vi "TimingTest.vi"() -> ()   [LabVIEW 2017]
uses:
  9d5949f9-07ca-45c6-940a-2e3a62ca42df.vi
  <vilib>/express/express analysis/Spectral/Block/exnSpectralBlock spectral measurements RMS poly.vi
  <vilib>/express/express analysis/Spectral/Block/exnSpectralBlock spectral measurements RMS DDT.vi
  <vilib>/express/express analysis/Spectral/XNode/ExpressSpectralMeasurementsBlockNode.xnode
panel:
  in  "100 Hz high-pass":bool
  out "Waveform Graph 2":dynamicdata(graph)
  out "Waveform Graph":dynamicdata(graph)
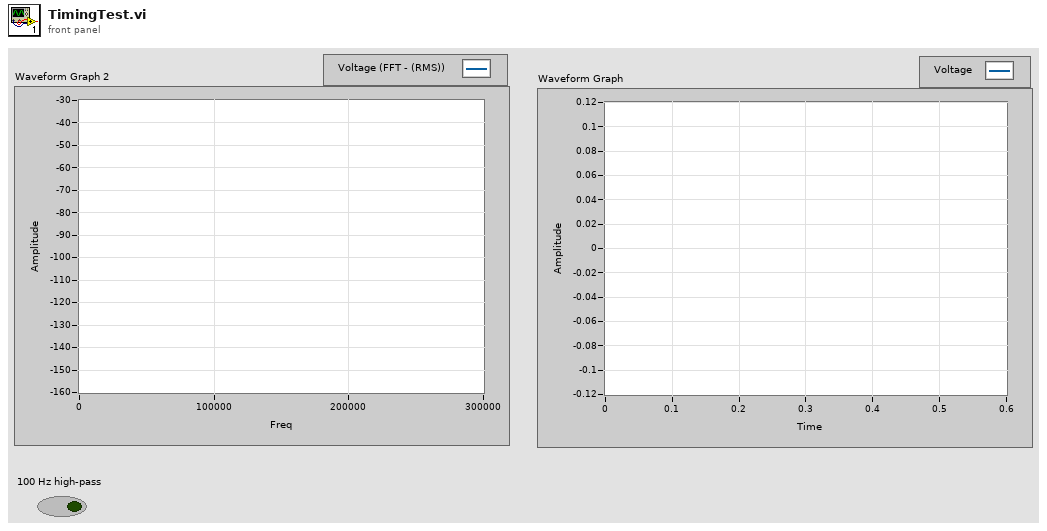
[diagram p1: front panel]
types:
  T1 = cluster{"averaging mode":u16, "weighting mode":u16, "number of averages":u32}
  T2 = cluster{"dB On (F)":bool, "unwrap phase (F)":bool, "convert to degree (F)":bool}
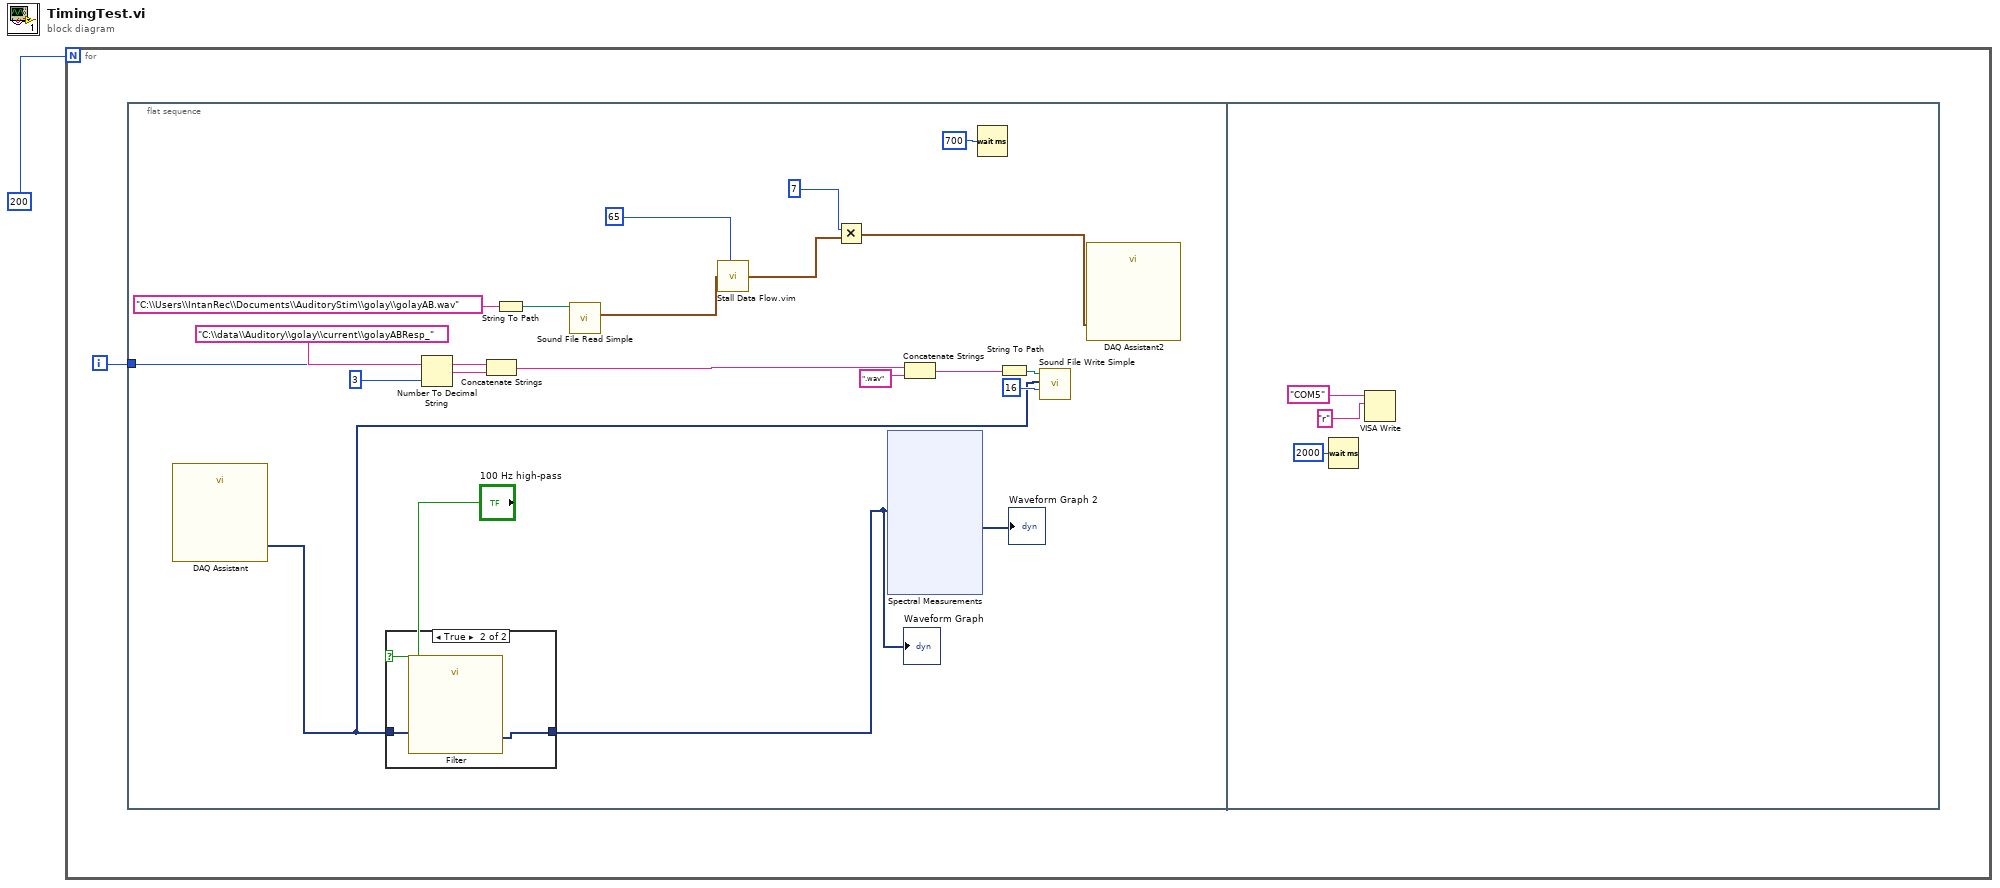
[diagram p0: block diagram]
diagram:
  n1 = for {
    N: 200 -> [_]
    i -> [w2]
    n2 = flat-sequence {
      tunnel: w2 -> [w19]
      frame #0 {
        n3 = call "DAQ Assistant"() -> ("data"=w7:dynamicdata)  [unwired: 17 in, 2 out]
        n4 = case shown="True" "100 Hz high-pass" {
          tunnel: w7 -> [w24 w26]
          tunnel: [w24 w25] -> w8
          frame False {
          }
          frame True {
            n5 = call "Filter"("Signal"=w26) -> ("Filtered Signal"=w25:dynamicdata)  [unwired: 9 in, 1 out]
          }
        }
        "Waveform Graph" <- w8
        n6 = Number To Decimal String(number=w19, width (-)=3) -> (decimal integer string=w17:string)
        n7 = Concatenate Strings("C:\\data\\Auditory\\golay\\current\\golayABResp_", w17) -> (w16:string)
        n8 = String To Path(string="C:\\Users\\IntanRec\\Documents\\AuditoryStim\\golay\\golayAB.wav") -> (path=w13:path)
        n9 = call <vilib>:"Sound File Read Simple.vi"("path"=w13) -> ("data"=w10:waveform(dbl)[])  [unwired: 7 in, 3 out]
        n10 = call "Stall Data Flow.vim"("value in"=w10, "milliseconds to wait"=65) -> ("value out"=w5:waveform(dbl)[])  [unwired: 1 out]
        n11 = Multiply(x=7, y=w5) -> (x*y=w3:waveform(dbl)[])
        n12 = xnode "Spectral Measurements"("Signals"=w8) -> ("FFT - (RMS)"=→"Waveform Graph 2":dynamicdata)  [unwired: 1 in, 2 out]
        n13 = Concatenate Strings(w16, ".wav") -> (w14:string)
        n14 = Wait (ms)(milliseconds to wait=700) -> ()  [unwired: 1 out]
        n15 = String To Path(string=w14) -> (path=w21:path)
        n16 = call <vilib>:"Sound File Write Simple.vi"("bits per sample"=16, "data"=w7, "path"=w21) -> ()  [unwired: 7 in, 2 out]
        n17 = call "DAQ Assistant2"("data"=w3) -> ()  [unwired: 17 in, 2 out]
      }
      frame #1 {
        n18 = Wait (ms)(milliseconds to wait=2000) -> ()  [unwired: 1 out]
        n19 = VISA Write(VISA resource name="COM5", write buffer="r") -> ()  [unwired: 1 in, 3 out]
      }
    }
  }
